vi "Test Submit.vi"(10 "Export in":refnum<class "Export.lvclass">, 11 "Commit in":refnum<class "Commit.lvclass">) -> (2 "Ready for Submit":bool, 3 "Commit out":refnum<class "Commit.lvclass">)   [LabVIEW 2017, in "CL_G3_VIComponentBuilder.lvlib" / "Commit.lvclass"]
doc: "Performs tests in order to ensure a successfull submission."
uses:
  Commit.lvclass
  Exports/Exports/Export.lvclass
  Commit.lvclass/Commit.ctl
  Accessors/Read Commit Operation Errors.vi
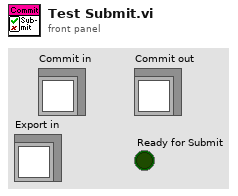
[diagram p1: front panel]
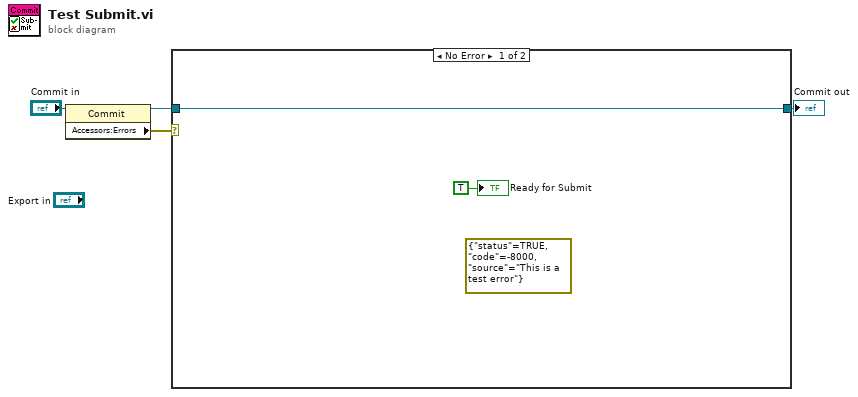
[diagram p0: block diagram]
diagram:
  n1 = property class="Commit"(reference="Commit in") -> (reference out=w2:refnum<class "Commit.lvclass">, "Accessors:Errors"=w1:errorcluster)  [unwired: 1 in, 1 out]
  n2 = case shown="No Error" w1 {
    tunnel: [w6 w7] -> w4
    tunnel: w2 -> [w6 w7]
    frame No Error {
      (unwired) errorcluster {"status"=TRUE, "code"=-8000, "source"="This is a test error"} ("error IO")
      "Ready for Submit" <- TRUE ("Boolean")
    }
    frame Error {
    }
  }
  "Commit out" <- w4
